vi "CRYPlot Wave Graph Preview.vi"(10 "sOption":string, 11 "Graph VI Ref":refnum<vi>) -> ()   [LabVIEW 2013]
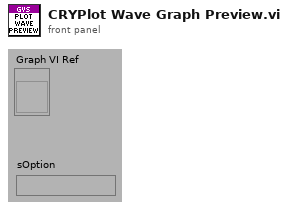
[diagram p1: front panel]
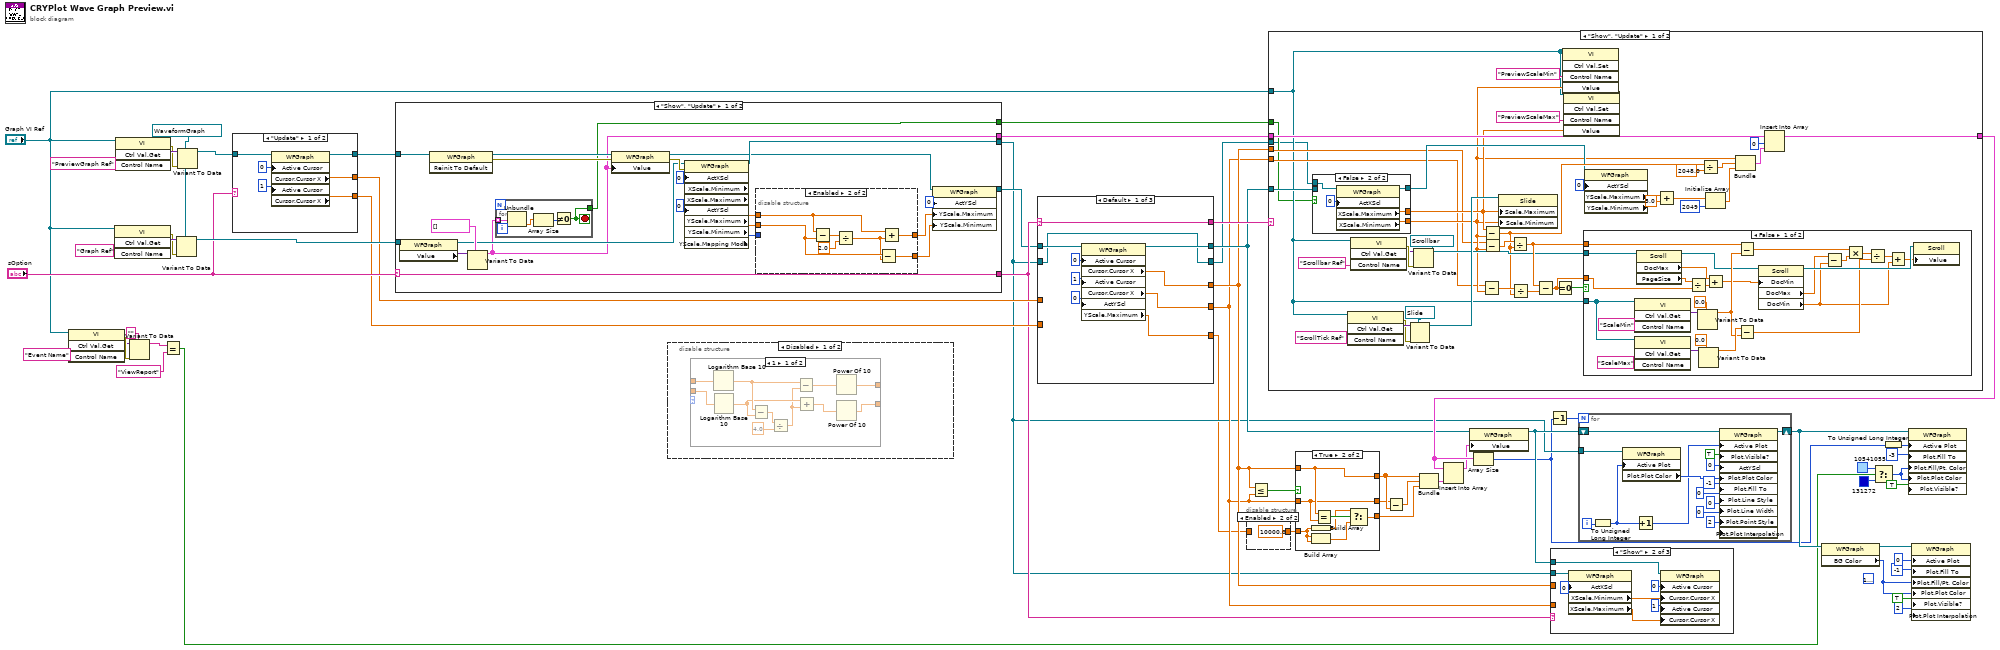
[diagram p0: block diagram]
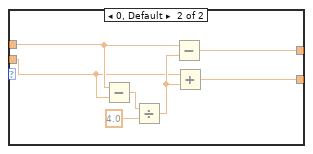
[diagram p3: hidden frame]
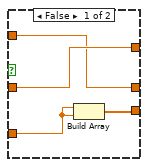
[diagram p5: hidden frame]
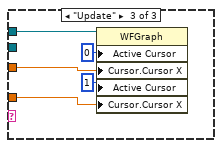
[diagram p8: hidden frame]
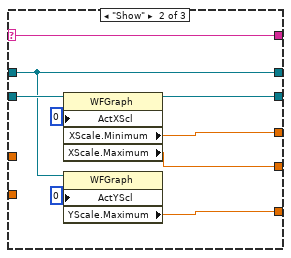
[diagram p9: hidden frame]
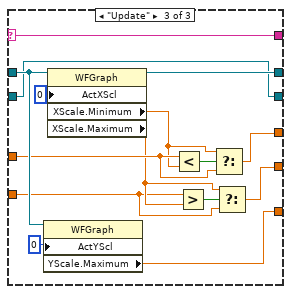
[diagram p10: hidden frame]
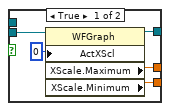
[diagram p11: hidden frame]
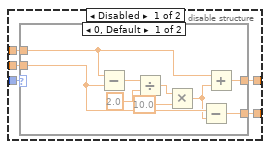
[diagram p14: hidden frame]
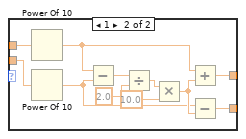
[diagram p15: hidden frame]
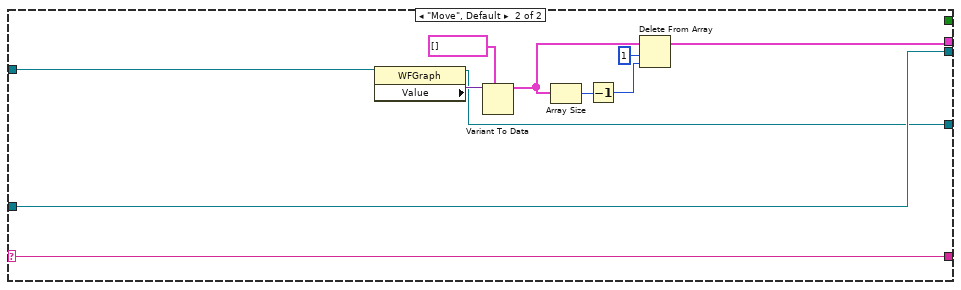
[diagram p16: hidden frame]
diagram:
  (unwired) u32 16777226
  w50 = refnum<vi> refnum ("Legend Ref")
  n1 = invoke class="VI" method="Ctrl Val.Get"(reference="Graph VI Ref", "Control Name"="Event Name") -> (error out=w9:errorcluster, "Get Control Value Variant"=w8:variant)  [unwired: 2 in, 2 out]
  n2 = invoke class="VI" method="Ctrl Val.Get"(reference="Graph VI Ref", "Control Name"="Graph Ref") -> (error out=w52:errorcluster, "Get Control Value Variant"=w53:variant)  [unwired: 2 in, 2 out]
  n3 = invoke class="VI" method="Ctrl Val.Get"(reference="Graph VI Ref", "Control Name"="PreviewGraph Ref") -> (error out=w56:errorcluster, "Get Control Value Variant"=w57:variant)  [unwired: 2 in, 2 out]
  n4 = Variant To Data(error in=w9, type="" ("Control Name"), Variant=w8) -> (data=w7:string)  [unwired: 1 out]
  n5 = Equal?(x=w7, y="ViewReport" ("Control Name")) -> (x = y?=w4:bool)
  n6 = Variant To Data(error in=w52, type=w50, Variant=w53) -> (data=w51:refnum<vi>)  [unwired: 1 out]
  n7 = Variant To Data(error in=w56, type=w50, Variant=w57) -> (data=w40:refnum<vi>)  [unwired: 1 out]
  n8 = case shown="\"Update\"" "sOption" {
    tunnel: [w63 w64] -> w38
    tunnel: [w62 _] -> w36
    tunnel: [w61 _] -> w37
    tunnel: w40 -> [w58 w64]
    frame "Update" {
      n9 = property on="Property Node" class="WFGraph"(reference=w58, "Active Cursor"=u32 0, "Active Cursor"=u32 1) -> (reference out=w63:refnum<vi>, "Cursor.Cursor X"=w61:dbl, "Cursor.Cursor X"=w62:dbl)  [unwired: 1 in, 1 out]
    }
    frame "Show", Default {
    }
  }
  n10 = case shown="\"Show\", \"Update\"" "sOption" {
    selector: "sOption" -> [w76 w123]
    tunnel: w38 -> [w86 w125]
    tunnel: w51 -> [w80 w133]
    tunnel: [w83 w124] -> w33
    tunnel: [w75 w133] -> w28
    tunnel: [w67 w126] -> w49
    tunnel: [w76 w123] -> w35
    tunnel: [w66 _] -> w15
    frame "Show", "Update" {
      n11 = property class="WFGraph"(reference=w80) -> (reference out=w74:refnum<vi>, "Value"=w81:variant)  [unwired: 1 in, 1 out]
      n12 = invoke class="WFGraph" method="Reinit To Default"(reference=w86) -> (reference out=w79:refnum<vi>, error out=w77:errorcluster)  [unwired: 2 in, 1 out]
      n13 = Variant To Data(type=cluster{"xo":dbl, "dx":dbl, dbl[]}[] [] ("appended array"), Variant=w81) -> (data=w67:cluster{"xo":dbl, "dx":dbl, dbl[]}[])  [unwired: 1 in, 1 out]
      n14 = for {
        tunnel: w67 -> [w122] mode=indexing
        tunnel: [w120] -> w66
        stop <- w120 stop-if-true
        n15 = Unbundle(w122) -> (w119:dbl[])  [unwired: 2 out]
        n16 = Array Size(array=w119) -> (size(s)=w121:i32)
        n17 = Not Equal To 0?(x=w121) -> (x != 0?=w120:bool)
      }
      n18 = property class="WFGraph"(reference=w79, error in=w77, "Value"=w67) -> (reference out=w69:refnum<vi>, error out=w78:errorcluster)
      n19 = property on="Property Node" class="WFGraph" props=["ActXScl", "XScale", "Minimum", "XScale", "Maximum", "ActYScl", "YScale", "Maximum", "YScale", "Minimum", "YScale", "Mapping Mode"](reference=w74, error in=w78, "ActXScl"=0 ("Active Y Scale"), "ActYScl"=0 ("Active Y Scale")) -> (reference out=w75:refnum<vi>, "YScale.Maximum"=w72:dbl, "YScale.Minimum"=w71:dbl, "YScale.Mapping Mode"=w65:u8)  [unwired: 3 out]
      n20 = disable-structure shown="Enabled" {
        disable-tunnel: [w91 w118] -> w73
        disable-tunnel: w72 -> [w90 w117]
        disable-tunnel: w71 -> [w89 w116]
        disable-tunnel: [w88 w115] -> w70
        disable-tunnel: w65 -> [w87 _]
        frame Disabled {
          n21 = case shown="0, Default" w87 {
            tunnel: [w98 w109] -> w91
            tunnel: w90 -> [w97 w104]
            tunnel: w89 -> [w96 w103]
            tunnel: [w95 w108] -> w88
            frame 0, Default {
              n22 = Subtract(x=w97, y=w96) -> (x-y=w100:dbl)
              n23 = Divide(x=w100, y=2.0) -> (x/y=w94:dbl)
              n24 = Multiply(x=w94, y=10.0) -> (x*y=w92:dbl)
              n25 = Subtract(x=w96, y=w92) -> (x-y=w95:dbl)
              n26 = Add(x=w97, y=w92) -> (x+y=w98:dbl)
            }
            frame 1 {
              n27 = Power Of 10(x=w104) -> (10^x=w102:dbl)
              n28 = Power Of 10(x=w103) -> (10^x=w101:dbl)
              n29 = Subtract(x=w102, y=w101) -> (x-y=w111:dbl)
              n30 = Divide(x=w111, y=2.0) -> (x/y=w107:dbl)
              n31 = Multiply(x=w107, y=10.0) -> (x*y=w105:dbl)
              n32 = Add(x=w102, y=w105) -> (x+y=w109:dbl)
              n33 = Subtract(x=w101, y=w105) -> (x-y=w108:dbl)
            }
          }
        }
        frame Enabled {
          n34 = Subtract(x=w117, y=w116) -> (x-y=w114:dbl)
          n35 = Divide(x=w114, y=2.0) -> (x/y=w112:dbl)
          n36 = Subtract(x=w116, y=w112) -> (x-y=w115:dbl)
          n37 = Add(x=w117, y=w112) -> (x+y=w118:dbl)
        }
      }
      n38 = property on="Property Node" class="WFGraph"(reference=w69, "ActYScl"=0 ("Active Y Scale"), "YScale.Maximum"=w73, "YScale.Minimum"=w70) -> (reference out=w83:refnum<vi>)  [unwired: 1 in, 1 out]
    }
    frame "Move", Default {
      n39 = property class="WFGraph"(reference=w125) -> (reference out=w124:refnum<vi>, "Value"=w131:variant)  [unwired: 1 in, 1 out]
      n40 = Variant To Data(type=cluster{"xo":dbl, "dx":dbl, dbl[]}[] [] ("appended array"), Variant=w131) -> (data=w129:cluster{"xo":dbl, "dx":dbl, dbl[]}[])  [unwired: 1 in, 1 out]
      n41 = Array Size(array=w129) -> (size(s)=w128:i32)
      n42 = Decrement(x=w128) -> (x-1=w127:i32)
      n43 = Delete From Array(array=w129, length=1, index=w127) -> (array with subset deleted=w126:cluster{"xo":dbl, "dx":dbl, dbl[]}[])  [unwired: 1 out]
    }
  }
  n44 = disable-structure shown="Disabled" {
    frame Disabled {
      n45 = case shown="1" {
        selector: _ -> [_ _]
        tunnel: _ -> [w143 w148]
        tunnel: _ -> [w141 w147]
        tunnel: [w135 w145] -> _
        tunnel: [w134 w146] -> _
        frame 1 {
          n46 = Logarithm Base 10(1:w143) -> (0:w144:dbl)
          n47 = Logarithm Base 10(1:w141) -> (0:w142:dbl)
          n48 = Subtract(x=w144, y=w142) -> (x-y=w138:dbl)
          n49 = Divide(x=w138, y=4.0) -> (x/y=w140:dbl)
          n50 = Subtract(x=w144, y=w140) -> (x-y=w137:dbl)
          n51 = Add(x=w142, y=w140) -> (x+y=w136:dbl)
          n52 = Power Of 10(x=w137) -> (10^x=w135:dbl)
          n53 = Power Of 10(x=w136) -> (10^x=w134:dbl)
        }
        frame 0, Default {
          n54 = Subtract(x=w148, y=w147) -> (x-y=w149:dbl)
          n55 = Divide(x=w149, y=4.0) -> (x/y=w151:dbl)
          n56 = Subtract(x=w148, y=w151) -> (x-y=w145:dbl)
          n57 = Add(x=w147, y=w151) -> (x+y=w146:dbl)
        }
      }
    }
    frame Enabled {
    }
  }
  n58 = case shown="Default" w35 {
    selector: w35 -> [w153 w162 w171]
    tunnel: [w161 w165 w183] -> w13
    tunnel: [w160 w164 w173] -> w32
    tunnel: [w158 w167 w174] -> w29
    tunnel: [w157 w168 w179] -> w30
    tunnel: w33 -> [w154 w164 w182]
    tunnel: w28 -> [w152 w169 w172]
    tunnel: w37 -> [_ _ w180]
    tunnel: w36 -> [_ _ w175]
    tunnel: [w152 w163 w172] -> w31
    tunnel: [w153 w162 w171] -> w34
    frame Default {
      n59 = property on="Property Node" class="WFGraph"(reference=w154, "Active Cursor"=u32 0, "Active Cursor"=u32 1, "ActYScl"=0 ("Active Y Scale")) -> (reference out=w160:refnum<vi>, "Cursor.Cursor X"=w157:dbl, "Cursor.Cursor X"=w158:dbl, "YScale.Maximum"=w161:dbl)  [unwired: 1 in, 1 out]
    }
    frame "Show" {
      n60 = property on="Property Node" class="WFGraph"(reference=w169, "ActXScl"=0 ("Active Y Scale")) -> (reference out=w163:refnum<vi>, "XScale.Minimum"=w168:dbl, "XScale.Maximum"=w167:dbl)  [unwired: 1 in, 1 out]
      n61 = property on="Property Node" class="WFGraph"(reference=w164, "ActYScl"=0 ("Active Y Scale")) -> ("YScale.Maximum"=w165:dbl)  [unwired: 1 in, 2 out]
    }
    frame "Update" {
      n62 = property on="Property Node" class="WFGraph"(reference=w182, "ActYScl"=0 ("Active Y Scale")) -> ("YScale.Maximum"=w183:dbl)  [unwired: 1 in, 2 out]
      n63 = property on="Property Node" class="WFGraph"(reference=w182, "ActXScl"=0 ("Active Y Scale")) -> (reference out=w173:refnum<vi>, "XScale.Minimum"=w178:dbl, "XScale.Maximum"=w176:dbl)  [unwired: 1 in, 1 out]
      n64 = Less?(x=w180, y=w178) -> (x < y?=w181:bool)
      n65 = Greater?(x=w175, y=w176) -> (0:w177:bool)
      n66 = Select(t=w178, s=w181, f=w180) -> (s? t:f=w179:dbl)
      n67 = Select(t=w176, s=w177, f=w175) -> (s? t:f=w174:dbl)
    }
  }
  n68 = disable-structure shown="Enabled" {
    disable-tunnel: w13 -> [w186 _]
    disable-tunnel: [w186 10000.0 ("YScale.Maximum")] -> w12
    frame Disabled {
    }
    frame Enabled {
    }
  }
  n69 = Less Or Equal?(x=w30, y=w29) -> (x <= y?=w19:bool)
  n70 = case shown="\"Show\", \"Update\"" w34 {
    tunnel: "Graph VI Ref" -> [w192 _]
    tunnel: w32 -> [w213 _]
    tunnel: w49 -> [w211 w264]
    tunnel: [w198 w264] -> w48
    tunnel: w31 -> [w188 _]
    tunnel: w30 -> [w194 _]
    tunnel: w29 -> [w193 _]
    tunnel: w15 -> [w189 _]
    frame "Show", "Update" {
      n71 = case shown="False" w189 {
        tunnel: w213 -> [w232 _]
        tunnel: [w231 w237] -> w207
        tunnel: [w230 w236] -> w203
        tunnel: [w229 w235] -> w200
        tunnel: w188 -> [_ w233]
        frame True {
          n72 = property on="Property Node" class="WFGraph"(reference=w232, "ActXScl"=0 ("Active X Scale")) -> (reference out=w231:refnum<vi>, "XScale.Maximum"=w230:dbl, "XScale.Minimum"=w229:dbl)  [unwired: 1 in, 1 out]
        }
        frame False {
          n73 = property on="Property Node" class="WFGraph"(reference=w233, "ActXScl"=0 ("Active X Scale")) -> (reference out=w237:refnum<vi>, "XScale.Maximum"=w236:dbl, "XScale.Minimum"=w235:dbl)  [unwired: 1 in, 1 out]
        }
      }
      n74 = invoke class="VI" method="Ctrl Val.Get"(reference=w192, "Control Name"="ScrollTick Ref") -> (error out=w220:errorcluster, "Get Control Value Variant"=w221:variant)  [unwired: 2 in, 2 out]
      n75 = invoke class="VI" method="Ctrl Val.Get"(reference=w192, "Control Name"="Scrollbar Ref") -> (error out=w215:errorcluster, "Get Control Value Variant"=w214:variant)  [unwired: 2 in, 2 out]
      n76 = Variant To Data(error in=w220, type=refnum<vi> refnum ("Legend Ref"), Variant=w221) -> (data=w223:refnum<vi>)  [unwired: 1 out]
      n77 = Variant To Data(error in=w215, type=refnum<vi> refnum ("Legend Ref"), Variant=w214) -> (data=w217:refnum<vi>)  [unwired: 1 out]
      n78 = Subtract(x=w193, y=w200) -> (x-y=w226:dbl)
      n79 = Subtract(x=w203, y=w200) -> (x-y=w209:dbl)
      n80 = Subtract(x=w194, y=w200) -> (x-y=w224:dbl)
      n81 = property on="Property Node" class="Slide"(reference=w223, "Scale.Maximum"=w203, "Scale.Minimum"=w200) -> ()  [unwired: 1 in, 2 out]
      n82 = Divide(x=w224, y=w209) -> (x/y=w225:dbl)
      n83 = Divide(x=w226, y=w209) -> (x/y=w227:dbl)
      n84 = Subtract(x=w225, y=w227) -> (x-y=w190:dbl)
      n85 = Equal To 0?(x=w190) -> (x = 0?=w191:bool)
      n86 = invoke class="VI" method="Ctrl Val.Set"(reference=w192, "Control Name"="PreviewScaleMin", "Value"=w200) -> ()  [unwired: 2 in, 5 out]
      n87 = invoke class="VI" method="Ctrl Val.Set"(reference=w192, "Control Name"="PreviewScaleMax", "Value"=w203) -> ()  [unwired: 2 in, 5 out]
      n88 = case shown="False" w191 {
        tunnel: w225 -> [w263 _]
        tunnel: w217 -> [w262 _]
        tunnel: w192 -> [w239 _]
        tunnel: w190 -> [w238 _]
        frame False {
          n89 = invoke class="VI" method="Ctrl Val.Get"(reference=w239, "Control Name"="ScaleMin") -> ("Get Control Value Variant"=w256:variant)  [unwired: 2 in, 3 out]
          n90 = invoke class="VI" method="Ctrl Val.Get"(reference=w239, "Control Name"="ScaleMax") -> ("Get Control Value Variant"=w259:variant)  [unwired: 2 in, 3 out]
          n91 = property on="Property Node" class="Scroll"(reference=w262) -> (reference out=w252:refnum<vi>, "DocMax"=w249:dbl, "PageSize"=w242:dbl)  [unwired: 1 in, 1 out]
          n92 = Divide(x=w242, y=w238) -> (x/y=w251:dbl)
          n93 = Variant To Data(type=0.0 ("X Scale.Range:Maximum"), Variant=w256) -> (data=w260:dbl)  [unwired: 1 in, 1 out]
          n94 = Variant To Data(type=0.0 ("X Scale.Range:Maximum"), Variant=w259) -> (data=w261:dbl)  [unwired: 1 in, 1 out]
          n95 = Add(x=w249, y=w251) -> (x+y=w250:dbl)
          n96 = Subtract(x=w263, y=w260) -> (x-y=w248:dbl)
          n97 = Subtract(x=w261, y=w260) -> (x-y=w245:dbl)
          n98 = property on="Property Node" class="Scroll"(reference=w252, "DocMin"=w250) -> (reference out=w253:refnum<vi>, "DocMax"=w240:dbl, "DocMin"=w241:dbl)  [unwired: 1 in, 1 out]
          n99 = Subtract(x=w240, y=w241) -> (x-y=w247:dbl)
          n100 = Multiply(x=w248, y=w247) -> (x*y=w246:dbl)
          n101 = Divide(x=w246, y=w245) -> (x/y=w244:dbl)
          n102 = Add(x=w244, y=w241) -> (x+y=w243:dbl)
          n103 = property on="Property Node" class="Scroll"(reference=w253, "Value"=w243) -> ()  [unwired: 1 in, 2 out]
        }
        frame True {
        }
      }
      n104 = property on="Property Node" class="WFGraph" props=["ActYScl", "YScale", "Maximum", "YScale", "Minimum"](reference=w207, "ActYScl"=0 ("Active Y Scale")) -> ("YScale.Maximum"=w196:dbl)  [unwired: 1 in, 3 out]
      n105 = Add(x=w196, y=5.0) -> (x+y=w206:dbl)
      n106 = Divide(x=w209, y=2048.0) -> (x/y=w201:dbl)
      n107 = Initialize Array(w206, 2049 ("dimension size")) -> (w202:dbl[])
      n108 = Bundle("XScale.Minimum"=w200, w201, w202) -> (w208:cluster{"XScale.Minimum":dbl, dbl, dbl[]})  [unwired: 1 in]
      n109 = Insert Into Array(array=w211, index=0, new element=w208) -> (w198:cluster{"xo":dbl, "dx":dbl, dbl[]}[])
    }
    frame Default {
    }
  }
  n110 = case shown="True" w19 {
    tunnel: [w268 w275] -> w27
    tunnel: w30 -> [w267 w275]
    tunnel: [w267 w274] -> w26
    tunnel: w29 -> [w268 w274]
    tunnel: w12 -> [w266 w270]
    tunnel: [w265 w271] -> w16
    frame False {
      n111 = Build Array(w266, w266) -> (w265:dbl[])
    }
    frame True {
      n112 = Build Array(w270) -> (w269:dbl[])
      n113 = Build Array(w270, w270) -> (w272:dbl[])
      n114 = Equal?(x=w275, y=w274) -> (x = y?=w273:bool)
      n115 = Select(t=w269, s=w273, f=w272) -> (s? t:f=w271:dbl[])
    }
  }
  n116 = Subtract(x=w26, y=w27) -> (x-y=w24:dbl)
  n117 = Bundle("Cursor.Cursor X"=w27, w24, w16) -> (w25:cluster{"Cursor.Cursor X":dbl, dbl, dbl[]})  [unwired: 1 in]
  n118 = Insert Into Array(array=w48, new element=w25) -> (w20:cluster{"xo":dbl, "dx":dbl, dbl[]}[])  [unwired: 1 in]
  n119 = property class="WFGraph"(reference=w32, "Value"=w20) -> (reference out=w41:refnum<vi>)  [unwired: 1 in, 1 out]
  n120 = Array Size(array=w48) -> (size(s)=w18:i32)
  n121 = Decrement(x=w18) -> (x-1=w17:i32)
  n122 = case shown="\"Show\"" w35 {
    tunnel: w41 -> [_ w277 w285]
    tunnel: w28 -> [_ w276 _]
    tunnel: w30 -> [_ _ w284]
    tunnel: w29 -> [_ _ w283]
    frame Default {
    }
    frame "Show" {
      n123 = property on="Property Node" class="WFGraph"(reference=w276, "ActXScl"=0 ("Active Y Scale")) -> ("XScale.Minimum"=w281:dbl, "XScale.Maximum"=w282:dbl)  [unwired: 1 in, 2 out]
      n124 = property on="Property Node" class="WFGraph"(reference=w277, "Active Cursor"=u32 0, "Cursor.Cursor X"=w281, "Active Cursor"=u32 1, "Cursor.Cursor X"=w282) -> ()  [unwired: 1 in, 2 out]
    }
    frame "Update" {
      n125 = property on="Property Node" class="WFGraph"(reference=w285, "Active Cursor"=u32 0, "Cursor.Cursor X"=w284, "Active Cursor"=u32 1, "Cursor.Cursor X"=w283) -> ()  [unwired: 1 in, 2 out]
    }
  }
  n126 = for {
    N: w17 -> [_]
    shift-right: [w292] -> w42
    shift-left: w41 -> [w293]
    tunnel: w28 -> [w290]
    i -> [w294]
    n127 = To Unsigned Long Integer(number=w294) -> (unsigned 32bit integer=w289:u32)
    n128 = property class="WFGraph"(reference=w290, "Active Plot"=w289) -> ("Plot.Plot Color"=w291:u32)  [unwired: 1 in, 2 out]
    n129 = Increment(x=w289) -> (x+1=w288:u32)
    n130 = property class="WFGraph"(reference=w293, "Active Plot"=w288, "Plot.Visible?"=TRUE ("Plot.Visible"), "ActYScl"=0 ("Active Y Scale"), "Plot.Plot Color"=w291, "Plot.Fill To"=i16 -1, "Plot.Line Style"=u8 0, "Plot.Line Width"=u8 0, "Plot.Point Style"=u8 0, "Plot.Plot Interpolation"=u8 2) -> (reference out=w292:refnum<vi>)  [unwired: 1 in, 1 out]
  }
  n131 = property on="Property Node" class="WFGraph"(reference=w42) -> (reference out=w43:refnum<vi>, "BG Color"=w14:u32)  [unwired: 1 in, 1 out]
  n132 = Select(t=u32 10541055, s=w4, f=u32 131272) -> (s? t:f=w1:u32)
  n133 = To Unsigned Long Integer(number=w18) -> (unsigned 32bit integer=w23:u32)
  n134 = property on="Property Node" class="WFGraph"(reference=w42, "Active Plot"=w23, "Plot.Fill To"=i16 -3, "Plot.Fill/Pt. Color"=w1, "Plot.Plot Color"=w1, "Plot.Visible?"=TRUE ("Plot.Visible")) -> ()  [unwired: 1 in, 2 out]
  n135 = property on="Property Node" class="WFGraph"(reference=w43, "Active Plot"=u32 0, "Plot.Fill To"=i16 -1, "Plot.Fill/Pt. Color"=w14, "Plot.Plot Color"=w14, "Plot.Visible?"=TRUE ("Plot.Visible"), "Plot.Plot Interpolation"=u8 2) -> ()  [unwired: 1 in, 2 out]
